vi "Test_ConstructTransport_InvalidRefnum_Error.vi"(8 "error in (no error)":errorcluster, 11 "TestCase in":refnum<class "TestListboxItemNamesBinding.lvclass">) -> (0 "error out":errorcluster, 3 "TestCase out":refnum<class "TestListboxItemNamesBinding.lvclass">)   [LabVIEW 2017, in "TestListboxItemNamesBinding.lvclass"]
uses:
  TestListboxItemNamesBinding.lvclass
  Source/Concrete/ListboxItemNamesBinding/ListboxItemNamesBinding.lvclass/ListboxItemNamesBinding.ctl
  <vilib>/Utility/error.llb/Error Cluster From Error Code.vi
  Source/Concrete/ListboxItemNamesBinding/ListboxItemNamesBinding.lvclass
panel:
  out "Return Error":errorcluster
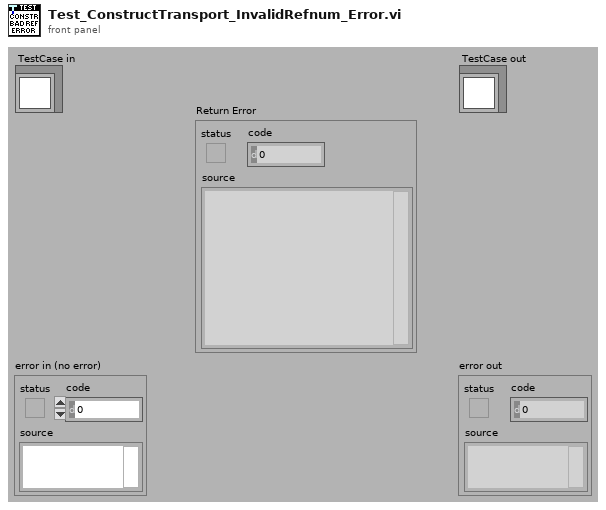
[diagram p1: front panel]
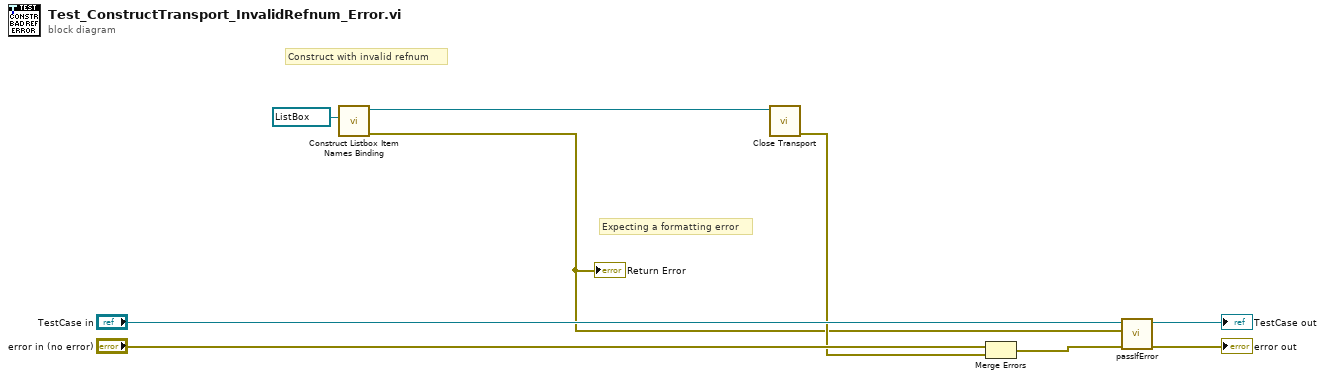
[diagram p0: block diagram]
diagram:
  # "Construct with invalid refnum"
  # "Expecting a formatting error"
  n1 = call "Construct Listbox Item Names Binding.vi"("LstBox Refnum"=refnum<vi> refnum) -> ("error out"=w2:errorcluster, "ListboxItemNamesBinding"=w3:refnum<class "ListboxItemNamesBinding.lvclass">)  [unwired: 9 in]
  "Return Error" <- w2
  n2 = call-dynamic "Close Transport.vi"("ITransport in"=w3) -> ("error out"=w4:errorcluster)  [unwired: 10 in]
  n3 = Merge Errors("error in (no error)", w4) -> (w5:errorcluster)
  n4 = call-dynamic "passIfError.vi"("error in (no error)"=w5, "error"=w2, "TestCase in"="TestCase in") -> ("error out"=→"error out":errorcluster, "TestCase out"=→"TestCase out":refnum<class "TestListboxItemNamesBinding.lvclass">)  [unwired: 7 in]
